vi "NI6008 LED Ctrl.vi"(8 "error in (no error)":errorcluster, 10 "On/Off":bool, 11 "Actor_NI6008 in":refnum<class "Actor_NI6008.lvclass">) -> (0 "error out":errorcluster, 3 "Actor_NI6008 out":refnum<class "Actor_NI6008.lvclass">)   [LabVIEW 2020, in "Actor_NI6008.lvlib" / "Actor_NI6008.lvclass"]
uses:
  Actor_NI6008.lvclass
  C:/Program Files/National Instruments/LabVIEW 2020/vi.lib/ActorFramework/Actor/Actor.lvclass
  <vilib>/ActorFramework/Actor/Actor.lvclass/Actor.ctl
  Actor_NI6008.lvclass/Actor_NI6008.ctl
  I_NI6008 Messages/NI6008 Status Report Msg/NI6008 Status Report Msg.lvclass/NI6008 Status Report Msg.ctl
  <vilib>/ActorFramework/Message Enqueuer/Message Enqueuer.lvclass/Message Enqueuer.ctl
  <vilib>/DAQmx/write.llb/DAQmx Write (Digital Bool 1Line 1Point).vi
  <vilib>/ActorFramework/Message Enqueuer/Enqueue.vi
  I_NI6008 Messages/NI6008 Status Report Msg/NI6008 Status Report Msg.lvclass
  C:/Program Files/National Instruments/LabVIEW 2020/vi.lib/ActorFramework/Message/Message.lvclass
  <vilib>/DAQmx/miscellaneous.llb/DAQmx Fill In Error Info.vi
  <vilib>/ActorFramework/Message Priority Queue/Priority Enqueue.vi
  <vilib>/ActorFramework/Actor/Actor.lvclass
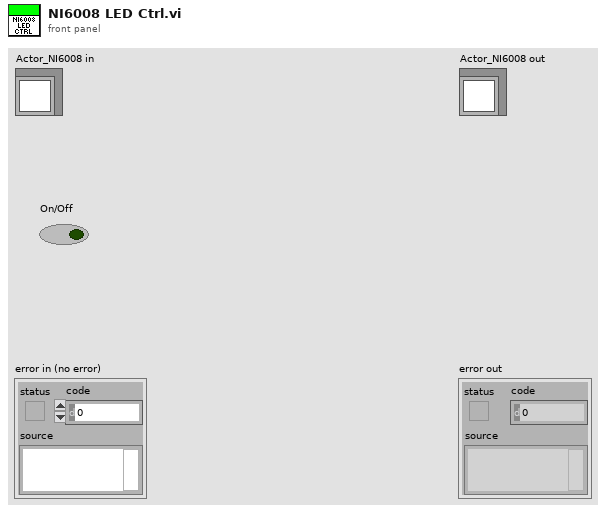
[diagram p1: front panel]
types:
  T1 = cluster{"Msg":string, "DO":bool[], "AI":dbl, "NI6008 Error":errorcluster}
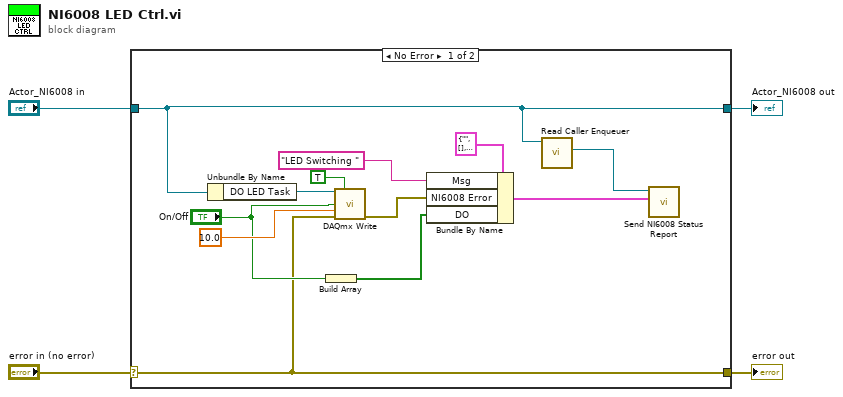
[diagram p0: block diagram]
diagram:
  n1 = case shown="No Error" "error in (no error)" {
    selector: "error in (no error)" -> [w5 w18]
    tunnel: [w5 w18] -> w3
    tunnel: [w6 w17] -> w1
    tunnel: "Actor_NI6008 in" -> [w6 w17]
    frame No Error {
      n2 = Unbundle By Name(w6) -> ("DO LED Task"=w12:refnum<k21>)
      n3 = Build Array("On/Off") -> (w9:bool[])
      n4 = call-poly <vilib>:"DAQmx Write.vi"("task/channels in"=w12, "auto start"=TRUE, "data"="On/Off", "timeout"=10.0, "error in"=w5) -> ("error out"=w8:errorcluster)  [unwired: 8 in, 2 out]
      n5 = Bundle By Name(cluster=T1 {"Msg"="", "DO"=[], "AI"=0.0, "NI6008 Error"={"status"=FALSE, "code"=0, "source"=""}} ("Data"), "Msg"="LED Switching ", "NI6008 Error"=w8, "DO"=w9) -> (w14:T1)
      n6 = call <vilib>:"Read Caller Enqueuer.vi"("Actor"=w6) -> ("Caller Enqueuer"=w13:refnum<class "Message Enqueuer.lvclass">)  [unwired: 10 in]
      n7 = call "Send NI6008 Status Report.vi"("Data"=w14, "Message Enqueuer"=w13) -> ()  [unwired: 8 in, 2 out]
    }
    frame Error {
    }
  }
  "error out" <- w3
  "Actor_NI6008 out" <- w1
